vi "Main.vi"() -> ()   [LabVIEW 2021]
panel:
  in  "加裝配備":enum16{"沒有", "電動座椅/電視音響"}(ring)
  in  "車身":enum16{"一般車身", "豪華加長車身"}(ring)
  in  "ま篮":enum16{"普通1600cc", "強力2400cc"}(ring)
  in  "底盤":enum16{"A型底盤", "B型底盤"}(ring)
  out "生產資訊":string
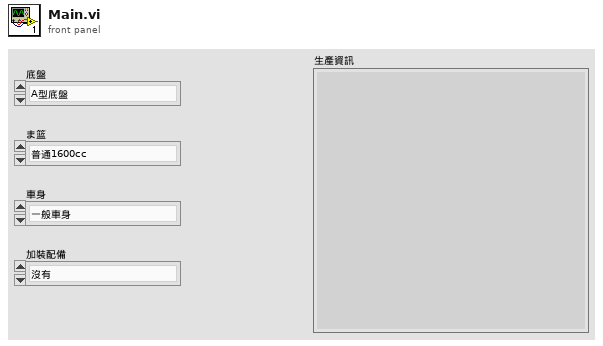
[diagram p1: front panel]
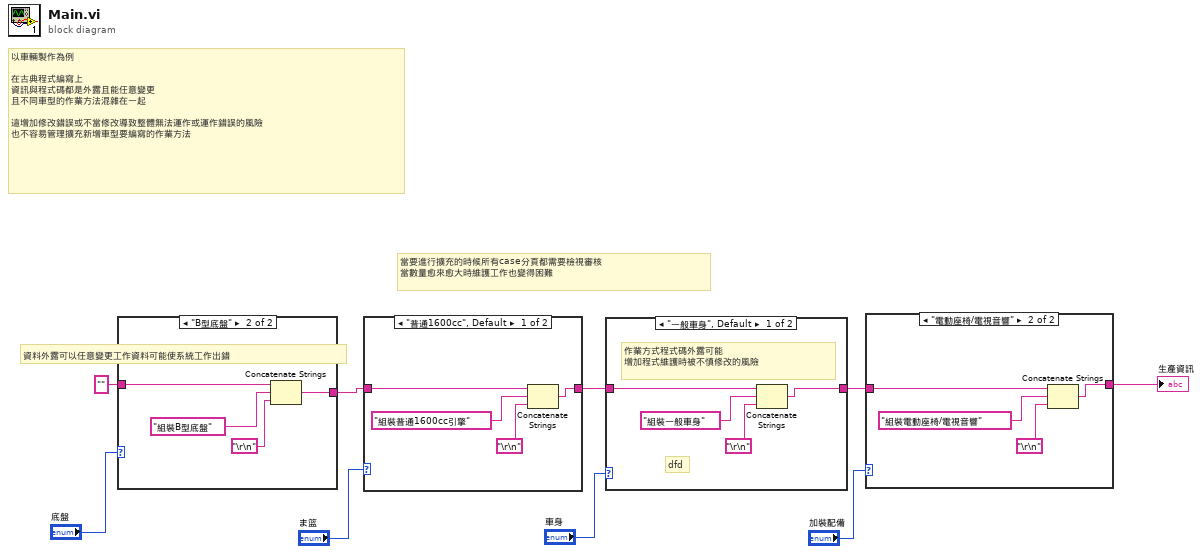
[diagram p0: block diagram]
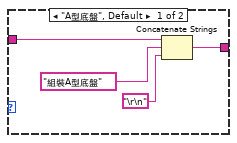
[diagram p2: hidden frame]
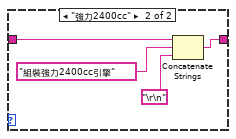
[diagram p3: hidden frame]
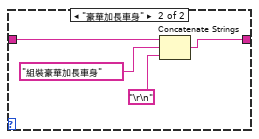
[diagram p4: hidden frame]
diagram:
  # "當要進行擴充的時候所有case分頁都需要檢視審核\n當數量愈來愈大時維護工作也變得困難"
  # "資料外露可以任意變更工作資料可能使系統工作出錯"
  # "以車輛製作為例\n\n在古典程式編寫上\n資訊與程式碼都是外露且能任意變更\n且不同車型的作業方法混雜在一起\n\n這增加修改錯誤或不當修改導致整體無法運作或運作錯誤的風險\n也不容易管理擴充新增車型要編寫的作業方法"
  n1 = case shown="\"B型底盤\"" "底盤" {
    tunnel: "" -> [w13 w17]
    tunnel: [w12 w16] -> w9
    frame "A型底盤", Default {
      n2 = Concatenate Strings(w13, "組裝A型底盤" ("string"), "\r\n") -> (w12:string)
    }
    frame "B型底盤" {
      n3 = Concatenate Strings(w17, "組裝B型底盤" ("string"), "\r\n") -> (w16:string)
    }
  }
  n4 = case shown="\"普通1600cc\", Default" "ま篮" {
    tunnel: w9 -> [w21 w25]
    tunnel: [w18 w22] -> w8
    frame "普通1600cc", Default {
      n5 = Concatenate Strings(w21, "組裝普通1600cc引擎" ("string"), "\r\n") -> (w18:string)
    }
    frame "強力2400cc" {
      n6 = Concatenate Strings(w25, "組裝強力2400cc引擎" ("string"), "\r\n") -> (w22:string)
    }
  }
  n7 = case shown="\"一般車身\", Default" "車身" {
    tunnel: w8 -> [w27 w31]
    tunnel: [w26 w30] -> w7
    frame "一般車身", Default {
      # "dfd"
      # "作業方式程式碼外露可能\n增加程式維護時被不慎修改的風險"
      n8 = Concatenate Strings(w27, "組裝一般車身" ("string"), "\r\n") -> (w26:string)
    }
    frame "豪華加長車身" {
      n9 = Concatenate Strings(w31, "組裝豪華加長車身" ("string"), "\r\n") -> (w30:string)
    }
  }
  n10 = case shown="\"電動座椅/電視音響\"" "加裝配備" {
    tunnel: w7 -> [w34 w36]
    tunnel: [w34 w35] -> w6
    frame "沒有", Default {
    }
    frame "電動座椅/電視音響" {
      n11 = Concatenate Strings(w36, "組裝電動座椅/電視音響" ("string"), "\r\n") -> (w35:string)
    }
  }
  "生產資訊" <- w6
